vi "FindingPatterns1.vi"() -> ()   [LabVIEW 2023]
uses:
  2024_11.lvclass
panel:
  out "x-y":u32
  out "Waveform Graph":dbl[](graph)
  out "Array 3":dbl[](array[numeric])
  out "spreadsheet string":string
  out "Array 2":i32[](array[numeric])
  out "Array":i32[](array[numeric])
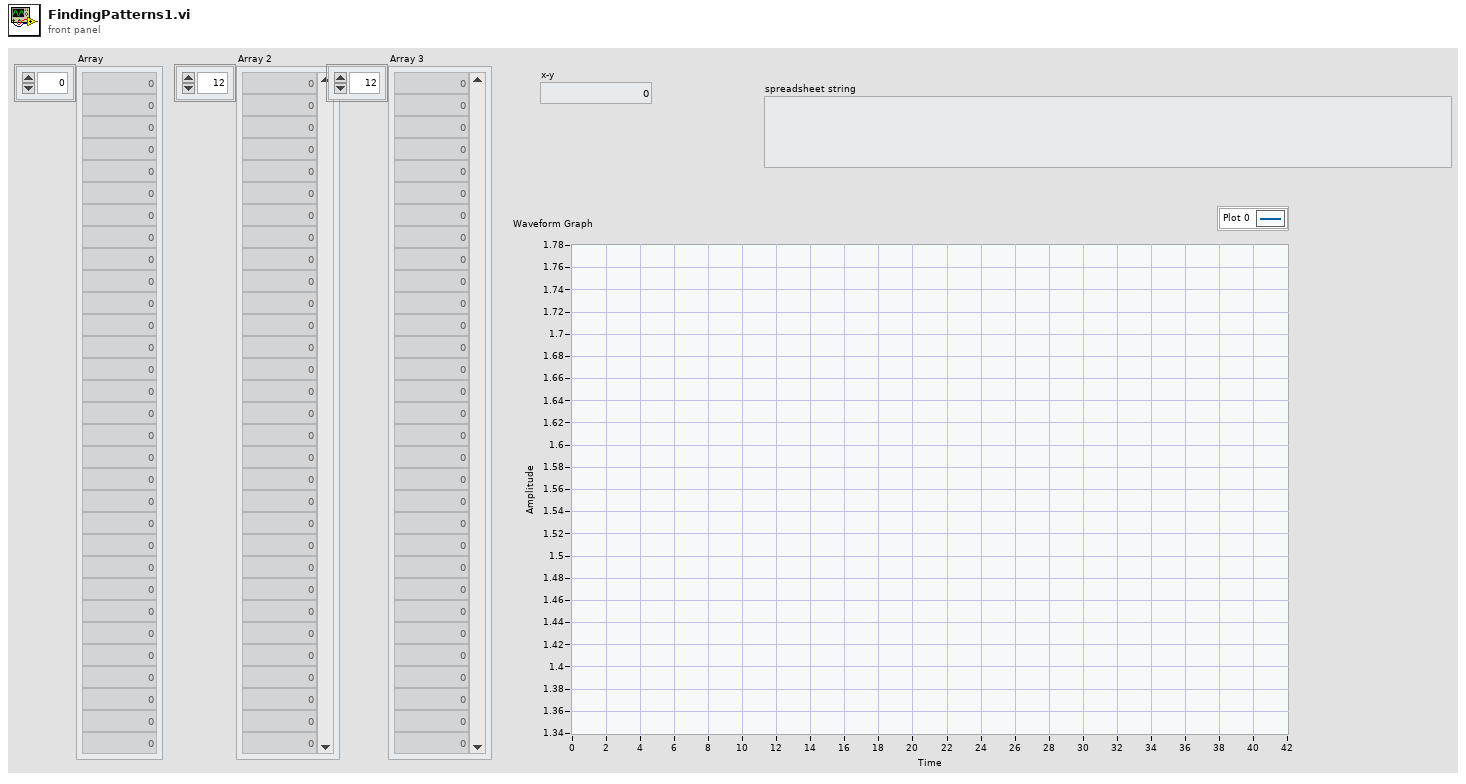
[diagram p1: front panel]
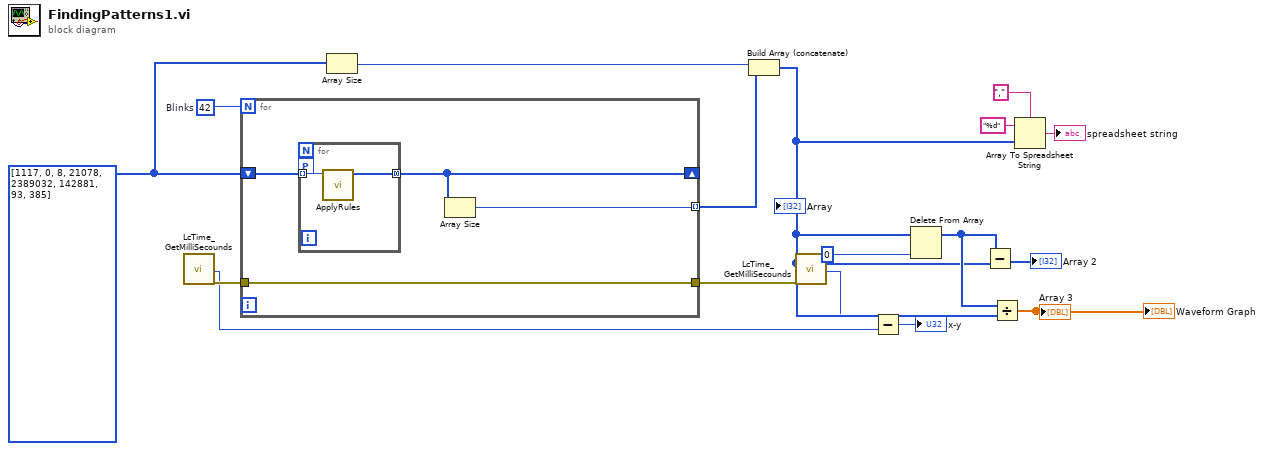
[diagram p0: block diagram]
diagram:
  w9 = u64[] [1117, 0, 8, 21078, 2389032, 142881, 93, 385] ("Numbers")
  w17 = 42  # Blinks
  n1 = call <userlib>:"LcTime_GetMilliSecounds.vi"() -> ("msValue"=w2:u32, "error out"=w15:errorcluster)  [unwired: 18 in]
  n2 = for {
    N: w17 -> [_]
    shift-right: [w19] -> _
    shift-left: w9 -> [w21]
    tunnel: [w20] -> w16
    tunnel: w15 -> [w20]
    tunnel: [w18] -> w7 mode=indexing
    n3 = for {
      tunnel: w21 -> [w23] mode=indexing
      tunnel: [w22] -> w19 mode=concatenating
      workers-P: _ -> [_]
      n4 = call "ApplyRules.vi"("Numeric"=w23) -> ("Array"=w22:u64[])  [unwired: 9 in, 1 out]
    }
    n5 = Array Size(array=w19) -> (size(s)=w18:i32)
  }
  n6 = Array Size(array=w9) -> (size(s)=w8:i32)
  n7 = Build Array (concatenate)(w8, w7) -> (w5:i32[])
  "Array" <- w5
  n8 = call <userlib>:"LcTime_GetMilliSecounds.vi"("error in (no error)"=w16) -> ("msValue"=w3:u32)  [unwired: 17 in, 1 out]
  n9 = Subtract(x=w3, y=w2) -> (x-y=→"x-y":u32)
  n10 = Delete From Array(array=w5, index=0) -> (array with subset deleted=w6:i32[])  [unwired: 1 in, 1 out]
  n11 = Subtract(x=w6, y=w5) -> (x-y=→"Array 2":i32[])
  n12 = Divide(x=w6, y=w5) -> (x/y=→"Array 3" →"Waveform Graph":dbl[])
  n13 = Array To Spreadsheet String(delimiter (Tab)=",", array=w5, 3:"%d" ("format string")) -> (spreadsheet string=→"spreadsheet string":string)
